vi "Charging_MICS Retry Count.vi"() -> ()   [LabVIEW 2020]
panel:
  in  "Retries":u8[](array[numeric])
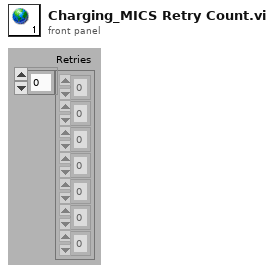
[diagram p1: front panel]
diagram:
